vi "svfa_Tone Estimation (magnitude).vi"(4 "linear/dB":enum16{"linear", "dB"}(ring), 6 "spectrum type":T1=enum."Power [Magnitude^2]", 8 "FFT size":i32, 9 "window size":i32, 10 "window":u16(ring) items=["None "=0, "Hanning"=1, "Hamming"=2, "Blackman-Harris"=3, "Exact Blackman"=4, "Blackman"=5, "Flat Top"=6, "4 Term B-Harris "=7, "7 Term B-Harris"=8, "Low Sidelobe"=9, "Force - Exponential"=10, "Gaussian"=62], 11 "three fingers":cluster{"f0":dbl, "df":dbl, "spectrum":dbl[]}={"f0"=0.0, "df"=1.0, "spectrum"=[]} {"spectrum" format="%.2f"; "df" format="%.2f"; "f0" format="%.2f"}) -> (3 "single tone info.":T2 {"phase [degree]" format="%.2f"; "amplitude" format="%.2f"; "frequency [Hz]" format="%.2f"})   [LabVIEW 2017]
doc: "This VI takes the three domainent FFT bins to apply the Newton-Raphson's root finding algorithm to determine the exact frequency, phase and amplitude.\nThe input is not necessary \"three fingers\", it could be two, four, or more."
uses:
  <vilib>/addons/_NISVFA/_Shared subVIs/Controls/svc_Spectrum Type.ctl
  <vilib>/addons/_NISVFA/_Spectrum Processing/subVIs/svfa_Tone Estimation Subroutine G(f) (magnitude).vi
  <vilib>/addons/_NISVFA/_Spectrum Processing/subVIs/svfa_Tone Estimation Subroutine G(f) (first derivative) (magnitude).vi
  <vilib>/addons/_NISVFA/_Spectrum Processing/subVIs/svfa_Initial Guess for Tone Estimation (magnitude).vi
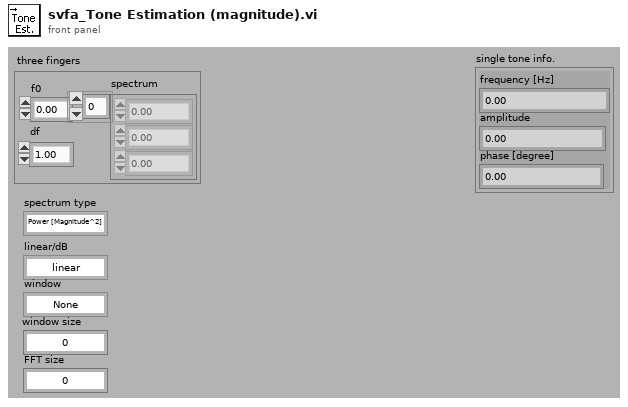
[diagram p1: front panel]
types:
  T1 = typedef "svc_Spectrum Type.ctl" = enum16{"FFT Spectrum [complex]", "Amplitude [Magnitude]", "Power [Magnitude^2]", "Cross Spectrum [complex]", "Frequency Response [Complex]"}
  T2 = cluster{"frequency [Hz]":dbl, "amplitude":dbl, "phase [degree]":dbl}
  T3 = cluster{"initial guess":dbl, "Amplitude":dbl, dbl}
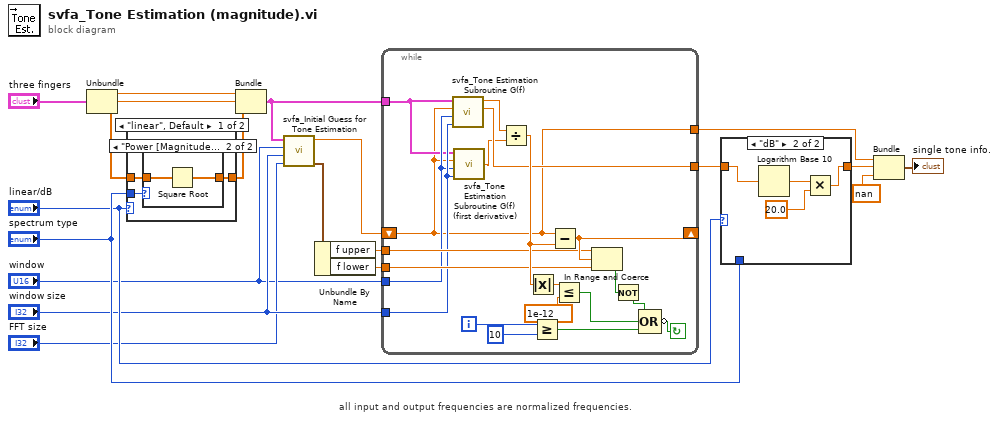
[diagram p0: block diagram]
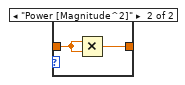
[diagram p3: hidden frame]
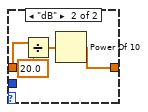
[diagram p5: hidden frame]
diagram:
  # "all input and output frequencies are normalized frequencies."
  n1 = Unbundle("three fingers") -> ("f0"=w6:dbl, "df"=w7:dbl, "spectrum"=w8:dbl[])
  n2 = case shown="\"linear\", Default" "linear/dB" {
    tunnel: w8 -> [w22 w30]
    tunnel: [w21 w27] -> w12
    tunnel: "spectrum type" -> [w23 _]
    frame "linear", Default {
      n3 = case shown="\"Power [Magnitude^2]\"" w23 {
        tunnel: [w24 w25] -> w21
        tunnel: w22 -> [w24 w26]
        frame "Amplitude [Magnitude]", Default {
        }
        frame "Power [Magnitude^2]" {
          n4 = Square Root(x=w26) -> (sqrt(x)=w25:dbl[])
        }
      }
    }
    frame "dB" {
      n5 = Divide(x=w30, y=20.0) -> (x/y=w28:dbl[])
      n6 = Power Of 10(x=w28) -> (10^x=w27:dbl[])
    }
  }
  n7 = Bundle("f0"=w6, "df"=w7, "spectrum"=w12) -> (w11:cluster{"f0":dbl, "df":dbl, "spectrum":dbl[]})  [unwired: 1 in]
  n8 = call-poly <vilib>:"svfa_Initial Guess for Tone Estimation.vi"("FFT size"="FFT size", "window size"="window size", "window"="window", "three fingers"=w11) -> ("range"=w15:cluster{"f upper":dbl, "f lower":dbl}, "initial guess"=w20:dbl)  [unwired: 6 in]
  n9 = Unbundle By Name(w15) -> ("f upper"=w14:dbl, "f lower"=w13:dbl)
  n10 = while {
    tunnel: w13 -> [w36]
    tunnel: w14 -> [w37]
    tunnel: "window size" -> [w35]
    tunnel: "window" -> [w34]
    tunnel: [w43] -> w17
    tunnel: [w31] -> w10
    shift-left: w20 -> [w31]
    shift-right: [w41] -> _
    tunnel: w11 -> [w33]
    i -> [w45]
    stop <- w47 continue-if-true
    n11 = call-poly <vilib>:"svfa_Tone Estimation Subroutine G(f).vi"("N (window length)"=w35, "window"=w34, "frequency"=w31, "three fingers"=w33) -> ("Amplitude"=w43:dbl, "G(f)"=w38:dbl)  [unwired: 2 in]
    n12 = call-poly <vilib>:"svfa_Tone Estimation Subroutine G(f) (first derivative).vi"("N (window length)"=w35, "window"=w34, "frequency"=w31, "three fingers"=w33) -> ("G'(f)"=w32:dbl)
    n13 = Divide(x=w38, y=w32) -> (x/y=w46:dbl)
    n14 = Absolute Value(x=w46) -> (abs(x)=w49:dbl)
    n15 = Greater Or Equal?(x=w45, y=10) -> (x >= y?=w48:bool)
    n16 = Subtract(x=w31, y=w46) -> (x-y=w41:dbl)
    n17 = Less Or Equal?(x=w49, y=1e-12) -> (x <= y?=w42:bool)
    n18 = In Range and Coerce(upper limit=w37, x=w41, lower limit=w36) -> (In Range?=w39:bool)  [unwired: 1 out]
    n19 = Not(x=w39) -> (.not. x?=w40:bool)
    n20 = Compound Arithmetic op=OR(w40, w42, w48) -> (invert w47:bool)
  }
  n21 = case shown="\"dB\"" "linear/dB" {
    tunnel: w17 -> [w52 w60]
    tunnel: [w51 w57] -> w16
    tunnel: "spectrum type" -> [w53 _]
    frame "linear", Default {
      n22 = case shown="\"Amplitude [Magnitude]\", Default" w53 {
        tunnel: [w54 w56] -> w51
        tunnel: w52 -> [w54 w55]
        frame "Amplitude [Magnitude]", Default {
        }
        frame "Power [Magnitude^2]" {
          n23 = Multiply(x=w55, y=w55) -> (x*y=w56:dbl)
        }
      }
    }
    frame "dB" {
      n24 = Logarithm Base 10(1:w60) -> (0:w59:dbl)
      n25 = Multiply(x=w59, y=20.0) -> (x*y=w57:dbl)
    }
  }
  n26 = Bundle("initial guess"=w10, "Amplitude"=w16, nan) -> (→"single tone info.":T3)  [unwired: 1 in]
